vi "player2.vi"(11 "Char":i16) -> (3 "f":i32)   [LabVIEW 2014]
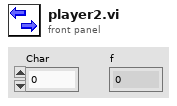
[diagram p1: front panel]
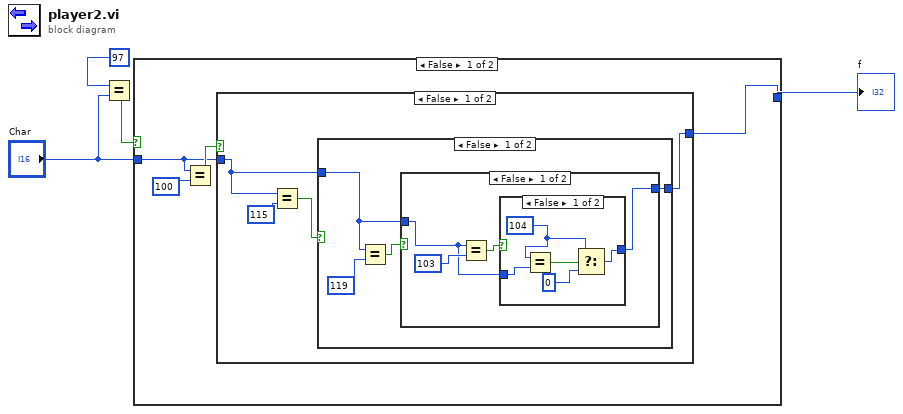
[diagram p0: block diagram]
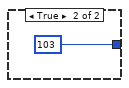
[diagram p2: hidden frame]
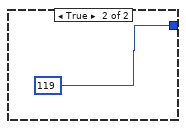
[diagram p3: hidden frame]
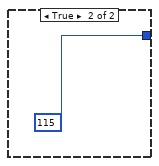
[diagram p4: hidden frame]
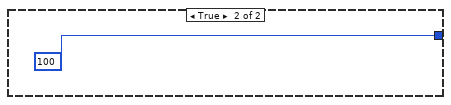
[diagram p5: hidden frame]
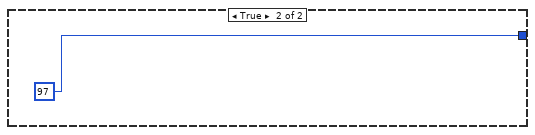
[diagram p6: hidden frame]
diagram:
  n1 = Equal?(x=97, y="Char") -> (x = y?=w2:bool)
  n2 = case shown="False" w2 {
    tunnel: "Char" -> [w5 _]
    tunnel: [w6 97] -> w4
    frame False {
      n3 = Equal?(x=w5, y=100) -> (x = y?=w7:bool)
      n4 = case shown="False" w7 {
        tunnel: [w10 100] -> w6
        tunnel: w5 -> [w9 _]
        frame False {
          n5 = Equal?(x=w9, y=115) -> (x = y?=w11:bool)
          n6 = case shown="False" w11 {
            tunnel: [w14 115] -> w10
            tunnel: w9 -> [w13 _]
            frame False {
              n7 = Equal?(x=w13, y=119) -> (x = y?=w15:bool)
              n8 = case shown="False" w15 {
                tunnel: [w17 119] -> w14
                tunnel: w13 -> [w18 _]
                frame False {
                  n9 = Equal?(x=w18, y=103) -> (x = y?=w20:bool)
                  n10 = case shown="False" w20 {
                    tunnel: [w23 103] -> w17
                    tunnel: w18 -> [w21 _]
                    frame False {
                      w24 = 104
                      n11 = Equal?(x=w24, y=w21) -> (x = y?=w25:bool)
                      n12 = Select(t=w24, s=w25, f=0) -> (s? t:f=w23:i32)
                    }
                    frame True {
                    }
                  }
                }
                frame True {
                }
              }
            }
            frame True {
            }
          }
        }
        frame True {
        }
      }
    }
    frame True {
    }
  }
  "f" <- w4
